vi "Configure_DMM.vi"(8 "error in (no error)":errorcluster, 10 "DMM_Configuration":T1={"Range"=10.0, "Measurement Type"=enum."DC Volts", "Resolution in Digits"=enum."5 1/2", "pin or relay names"=""} {"Range" format="%.2f"}, 11 "niDMM in":refnum<class "niDMM.lvclass">) -> (0 "error out":errorcluster, 3 "niDMM out":refnum<class "niDMM.lvclass">)   [LabVIEW 2020, in "niDMM.lvclass"]
uses:
  niDMM.lvclass
  DMM_Base/Typedef/DMM_Configuration.ctl
  <instrlib>/niDMM/nidmm.llb/niDMM Resolution in Digits.ctl
  <instrlib>/niDMM/nidmm.llb/niDMM Configure Measurement Digits.vi
  <vilib>/MeasurementLink/MeasurementLink niDMM/MeasurementLink niDMM.lvlib
  DMM_Base/DMM_Base.lvclass
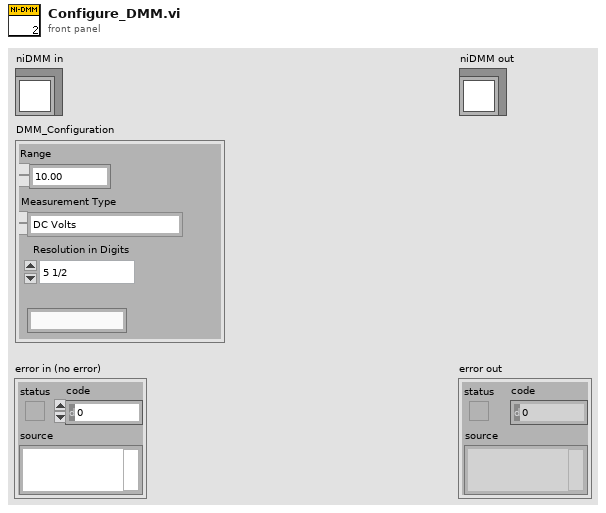
[diagram p1: front panel]
types:
  T1 = typedef "DMM_Base.lvclass/DMM_Configuration.ctl" = cluster{"Range":dbl, "Measurement Type":enum32{"DC Volts", "AC Volts", "DC Current", "AC Current", "2-wire Resistance", "4-wire Resistance", "Diode", "Frequency", "Period", "AC Volts DC Coupled", "Capacitance", "Inductance", "Temperature"}, "Resolution in Digits":enum32{"3 1/2", "4 1/2", "5 1/2", "6 1/2", "7 1/2"}, "pin or relay names":string}
  T2 = enum32{"3 1/2", "4 1/2", "5 1/2", "6 1/2", "7 1/2"}
  T3 = enum32{"DC Volts", "AC Volts", "DC Current", "AC Current", "2-wire Resistance", "4-wire Resistance", "Diode", "Frequency", "Period", "AC Volts DC Coupled", "Capacitance", "Inductance", "Temperature"}
  T4 = typedef "MeasurementLink niDMM.lvlib/Connection with Session.ctl" = cluster{"connection":T5, "session":refnum<k15>}
  T5 = typedef "MeasurementLink Session Management V1.lvlib/Session Reservation.lvclass/Connection.ctl" = cluster{"pin or relay name":string, "site":i32, "instrument type id":string, "channel":string}
  T6 = typedef "niDMM Resolution in Digits.ctl" = dbl
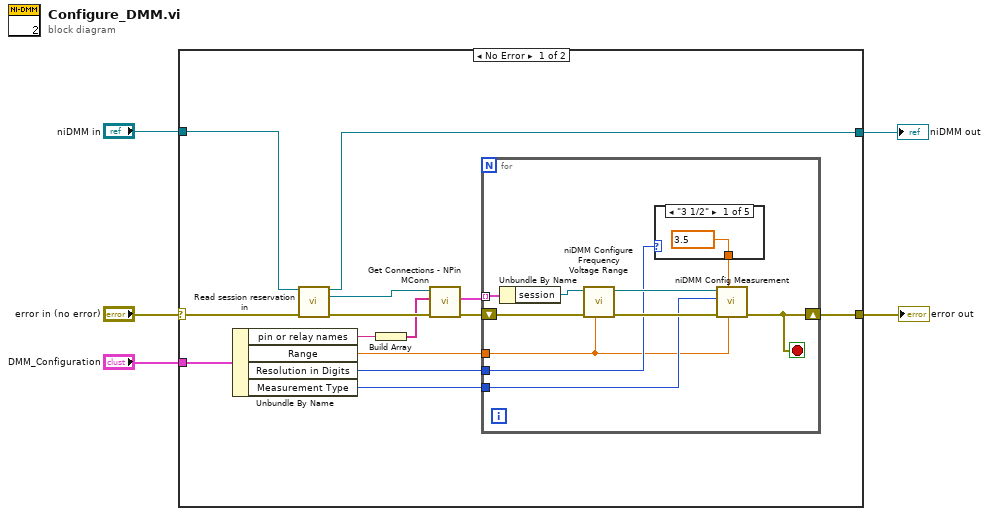
[diagram p0: block diagram]
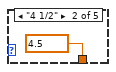
[diagram p2: hidden frame]
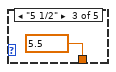
[diagram p3: hidden frame]
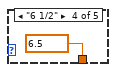
[diagram p4: hidden frame]
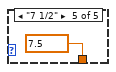
[diagram p5: hidden frame]
diagram:
  n1 = case shown="No Error" "error in (no error)" {
    selector: "error in (no error)" -> [w10 w35]
    tunnel: "DMM_Configuration" -> [w11 _]
    tunnel: "niDMM in" -> [w9 w36]
    tunnel: [w8 w36] -> w2
    tunnel: [w7 w35] -> w1
    frame No Error {
      n2 = Unbundle By Name(w11) -> ("pin or relay names"=w12:string, "Range"=w17:dbl, "Resolution in Digits"=w18:T2, "Measurement Type"=w19:T3)
      n3 = call-dynamic "Read session reservation in.vi"("AbstractDMM in"=w9, "error in (no error)"=w10) -> ("AbstractDMM out"=w8:refnum<class "niDMM.lvclass">, "MeasurementLink Session Management V1.lvlib:Session Reservation.lvclass"=w16:refnum<class "Session Reservation.lvclass">, "error out"=w15:errorcluster)  [unwired: 11 in]
      n4 = Build Array(w12) -> (w6:string[])
      n5 = call <vilib>:"Get Connections - NPin MConn.vi"("error in"=w15, "pin or relay names"=w6, "session reservation in"=w16) -> ("error out"=w14:errorcluster, "connections"=w13:T4[])  [unwired: 6 in, 1 out]
      n6 = for {
        tunnel: w19 -> [w26]
        tunnel: w18 -> [w25]
        tunnel: w17 -> [w24]
        shift-right: [w20] -> w7
        shift-left: w14 -> [w23]
        tunnel: w13 -> [w22] mode=indexing
        stop <- w20 stop-if-true
        n7 = Unbundle By Name(w22) -> ("session"=w21:refnum<k15>)
        n8 = call <instrlib>:"niDMM Configure Frequency Voltage Range.vi"("Frequency Voltage Range"=w24, "error in (no error)"=w23, "instrument handle"=w21) -> ("error out"=w29:errorcluster, "instrument handle out"=w28:refnum<k15>)  [unwired: 7 in]
        n9 = case shown="\"3 1/2\"" w25 {
          tunnel: [w30 w31 w32 w33 w34] -> w27
          frame "3 1/2" {
            w30 = T6 3.5 items=["3 1/2"=3.5, "4 1/2"=4.5, "5 1/2"=5.5, "6 1/2"=6.5, "7 1/2"=7.5] ("Resolution in Digits")
          }
          frame "4 1/2" {
            w31 = T6 4.5 items=["3 1/2"=3.5, "4 1/2"=4.5, "5 1/2"=5.5, "6 1/2"=6.5, "7 1/2"=7.5] ("Resolution in Digits")
          }
          frame "5 1/2" {
            w32 = T6 5.5 items=["3 1/2"=3.5, "4 1/2"=4.5, "5 1/2"=5.5, "6 1/2"=6.5, "7 1/2"=7.5] ("Resolution in Digits")
          }
          frame "6 1/2" {
            w33 = T6 6.5 items=["3 1/2"=3.5, "4 1/2"=4.5, "5 1/2"=5.5, "6 1/2"=6.5, "7 1/2"=7.5] ("Resolution in Digits")
          }
          frame "7 1/2" {
            w34 = T6 7.5 items=["3 1/2"=3.5, "4 1/2"=4.5, "5 1/2"=5.5, "6 1/2"=6.5, "7 1/2"=7.5] ("Resolution in Digits")
          }
        }
        n10 = call-poly <instrlib>:"niDMM Config Measurement.vi"("Range"=w24, "Resolution in Digits"=w27, "error in (no error)"=w29, "Function"=w26, "instrument handle"=w28) -> ("error out"=w20:errorcluster)  [unwired: 5 in, 1 out]
      }
    }
    frame Error {
    }
  }
  "error out" <- w1
  "niDMM out" <- w2
